vi "mod_Demodulate AM (DSB).vi"(0 "IQ data (complex)":cluster{"t0":dbl, "dt":dbl, "Y":cdb[]} {"Y" format="%.2f"; "dt" format="%.2f"; "t0" format="%.2f"}, 5 "modulation index":dbl=1.0 format="%.2f", 11 "error in (no error)":errorcluster, 12 "suppress carrier ?":bool) -> (4 "AM demodulated waveform":waveform(dbl), 6 "carrier amplitude":dbl format="%.2f", 15 "error out":errorcluster)   [LabVIEW 2020, in "niAMT.lvlib"]
doc: "Performs amplitude demodulation on the I-Q signal. This VI computes the magnitude of the complex I-Q data, subtracts the carrier wave amplitude, and then removes the carrier amplitude scaling from the I-Q signal to recover the information signal. The original information signal is returned in the <B>AM demodulated waveform</B> output."
uses:
  <vilib>/addons/Modulation/niAMT.lvlib
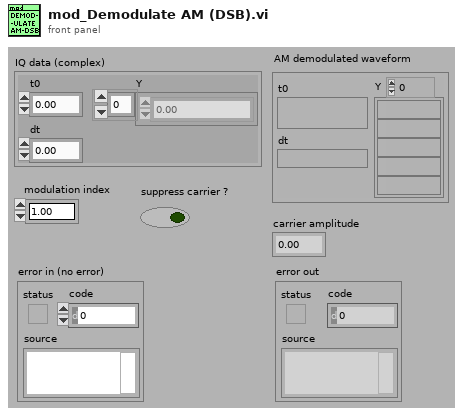
[diagram p1: front panel]
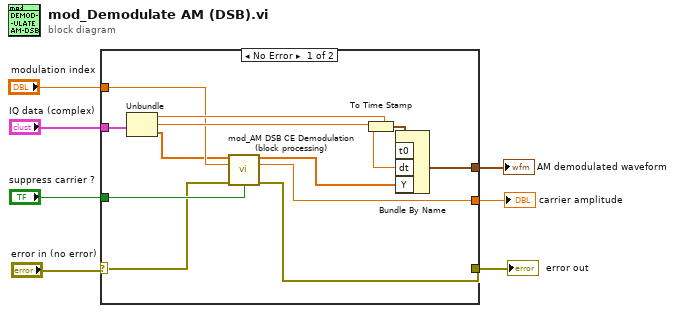
[diagram p0: block diagram]
diagram:
  n1 = case shown="No Error" "error in (no error)" {
    selector: "error in (no error)" -> [w12 w20]
    tunnel: [w11 w20] -> w7
    tunnel: [w19 _] -> w5
    tunnel: "IQ data (complex)" -> [w16 _]
    tunnel: "modulation index" -> [w14 _]
    tunnel: "suppress carrier ?" -> [w13 _]
    tunnel: [w10 _] -> w1
    frame No Error {
      n2 = Unbundle(w16) -> ("t0"=w18:dbl, "dt"=w17:dbl, "Y"=w9:cdb[])
      n3 = call <vilib>:"mod_AM DSB CE Demodulation (block processing).vi"("x"=w9, "modulation index"=w14, "error in (no error)"=w12, "suppress carrier ?"=w13) -> ("AM demod"=w8:dbl[], "carrier amplitude"=w10:dbl, "error out"=w11:errorcluster)  [unwired: 2 in, 7 out]
      n4 = To Time Stamp(1:w18) -> (0:w15:timestamp)
      n5 = Bundle By Name("t0"=w15, "dt"=w17, "Y"=w8) -> (w19:waveform(dbl))  [unwired: 1 out]
    }
    frame Error {
    }
  }
  "error out" <- w7
  "carrier amplitude" <- w1
  "AM demodulated waveform" <- w5
